vi "Compare pattern (SubVI).vi"(8 "error in":errorcluster, 9 "divider":sgl=1.6, 10 "Angle (degrees)":sgl format="%.2f", 11 "Pattern classes":i32[](array[numeric])) -> (0 "error out":errorcluster, 1 "Number of Matches":i32, 2 "Calibrated Matches":T1[](array[typedef]) {"Correlation Score" format="%.2f"; "Target Template Curve Score" format="%.2f"; "Template Target Curve Score" format="%.2f"; "Bounding Box"."y" format="%.2f"; "Bounding Box"."x" format="%.2f"; "Position"."y" format="%.2f"; "Position"."x" format="%.2f"; "Score" format="%.2f"; "Scale" format="%.2f"; "Angle" format="%.2f"; "Occlusion %" format="%.2f"}, 3 "Pattern":i32, 4 "pattern match":bool)   [LabVIEW 2017]
uses:
  <vilib>/vision/Pattern Matching.llb/IMAQ GM Match Report.ctl
  <vilib>/userdefined/High Color/IMAQdx.ctl
  <vilib>/vision/NI_Vision_Development_Module.lvlib
  <vilib>/vision/driver/NI_Vision_Acquisition_Software.lvlib
panel:
  out "x0":i32
  out "y0":i32
  in  "ROI":T2={"Global Rectangle"=[109, 72, 345, 284], "Contours"=[{"ID"=enum."External", "Type"=3, "Coordinates"=[109, 72, 345, 284]}]} {"Contours"."Type" items=["No Selection", "Point", "Line", "Rectangle", "Oval", "Polygon", "Freehand Region", "Annulus", "Unused2", "Unused3", "Broken Line", "Freehand Line", "Rotated Rectangle"]}
  out "Scale":sgl
  out "x1":i32
  out "y1":i32
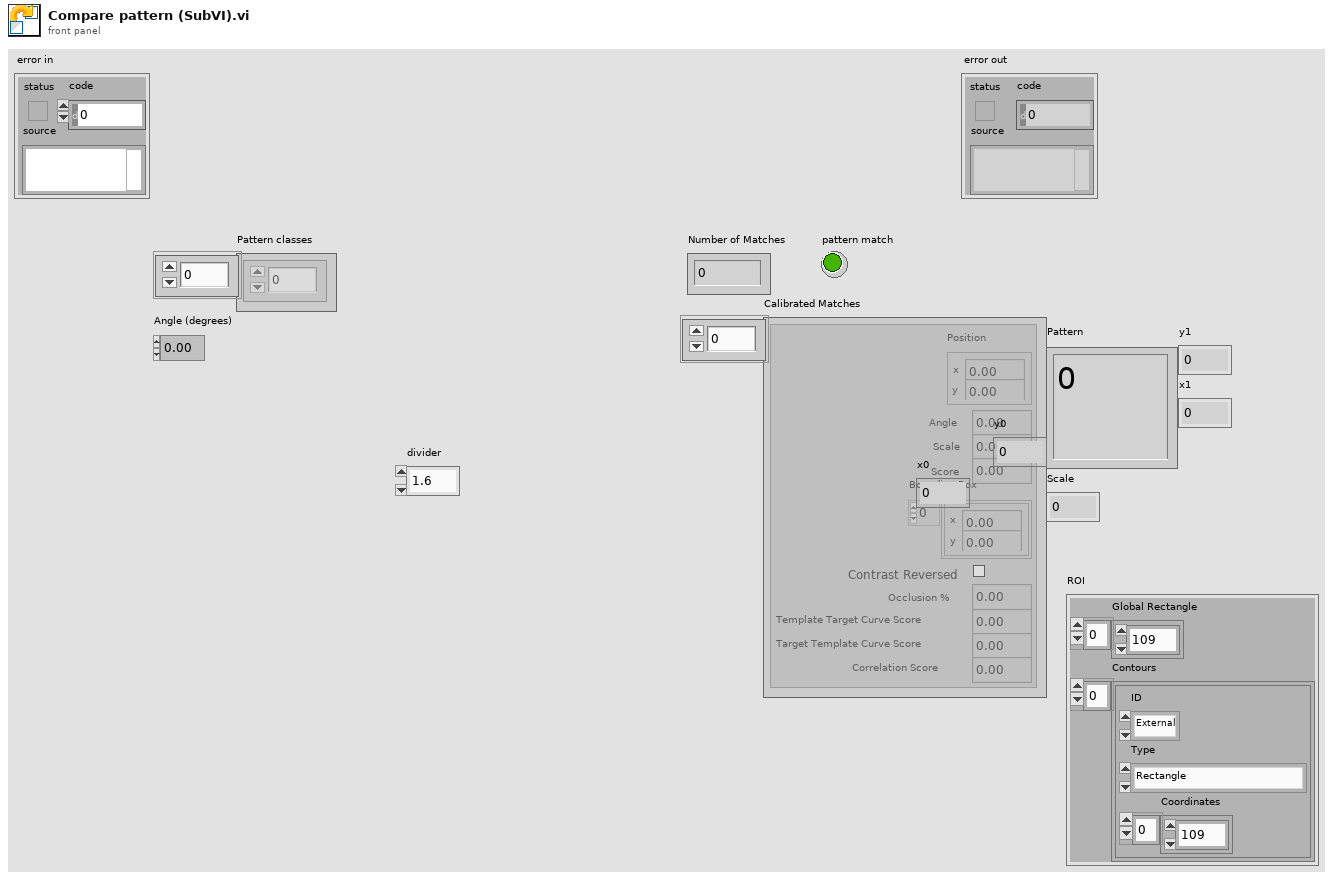
[diagram p1: front panel]
types:
  T1 = typedef "IMAQ GM Match Report.ctl" = cluster{"Position":cluster{"x":sgl, "y":sgl}, "Angle":sgl, "Scale":sgl, "Score":sgl, "Bounding Box":cluster{"x":sgl, "y":sgl}[], "Contrast Reversed":bool, "Occlusion %":sgl, "Template Target Curve Score":sgl, "Target Template Curve Score":sgl, "Correlation Score":sgl}
  T2 = cluster{"Global Rectangle":i32[], "Contours":cluster{"ID":enum32{"External", "Internal"}, "Type":u32, "Coordinates":i32[]}[]}
  T3 = typedef "IMAQdx.ctl" = refnum<k21>
  T4 = typedef "IMAQ Image.ctl" = refnum<image>
  T5 = cluster{"ID":enum32{"External", "Internal"}, "Type":u32, "Coordinates":i32[]}[]
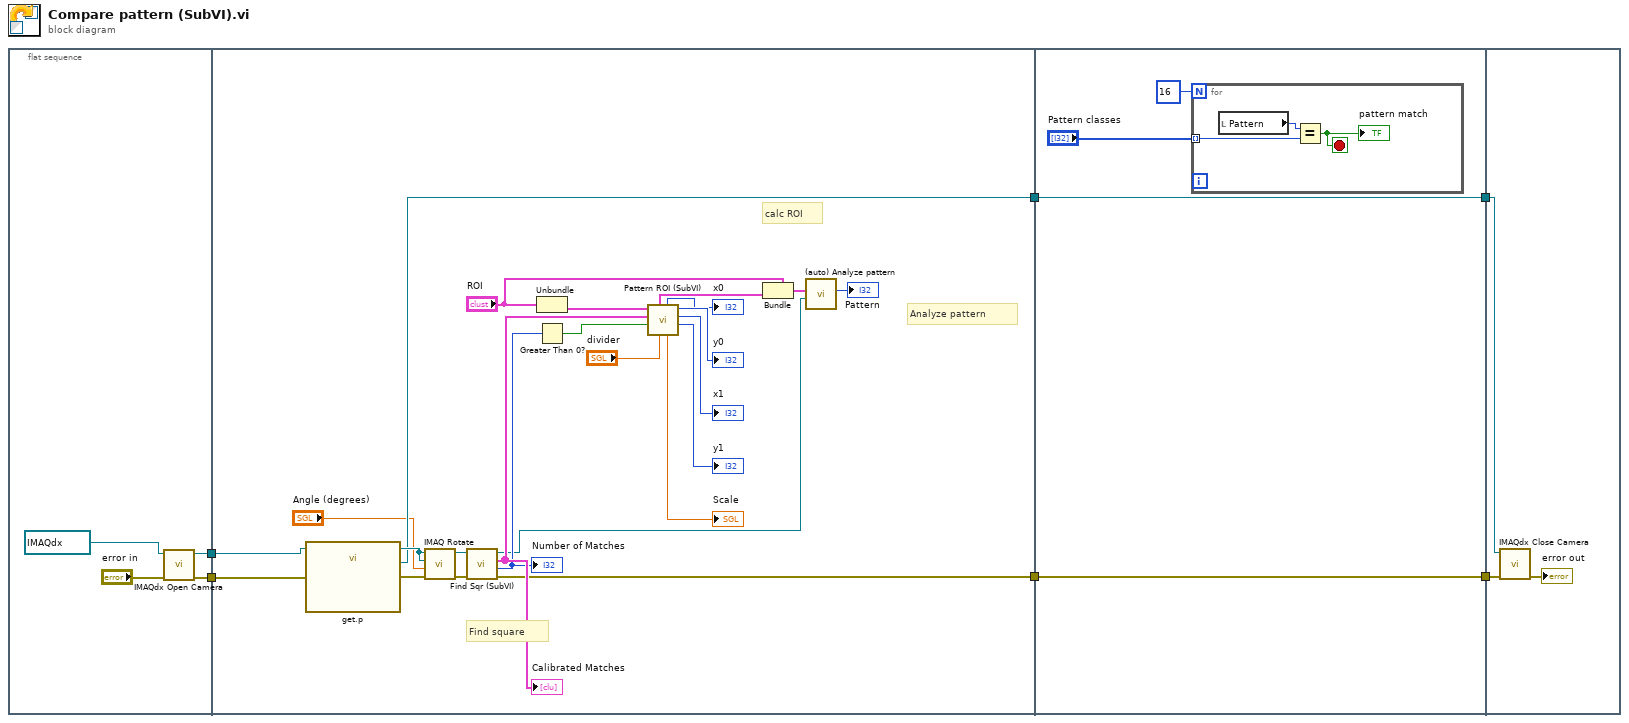
[diagram p0: block diagram]
diagram:
  n1 = flat-sequence {
    tunnel: [w8] -> w6
    tunnel: [w9] -> w5
    tunnel: w6 -> [w15]
    tunnel: w5 -> [w14]
    tunnel: [w13] -> w4
    tunnel: [w11] -> w2
    tunnel: w4 -> [w38]
    tunnel: [w38] -> w3
    tunnel: w2 -> [w35]
    tunnel: [w35] -> w1
    tunnel: w3 -> [w44]
    tunnel: w1 -> [w43]
    frame #0 {
      n2 = call <vilib>:"IMAQdx Open Camera.vi"("error in"="error in", "Session In"=T3 "cam0") -> ("error out"=w9:errorcluster, "Session Out"=w8:T3)  [unwired: 8 in]
    }
    frame #1 {
      # "calc ROI"
      # "Analyze pattern"
      # "Find square"
      n3 = call "get.p.vi"("Session in"=w15, "error in"=w14) -> ("Image Out"=w33:T4, "Session Out"=w13:T3, "error out"=w34:errorcluster)  [unwired: 23 in]
      n4 = call "IMAQ Rotate"("error in (no error)"=w34, "Angle (degrees)"="Angle (degrees)", "Image Dst"=w33, "Image Src"=w33) -> ("error out"=w31:errorcluster, "Image Dst Out"=w32:T4)  [unwired: 6 in]
      n5 = call "Find Sqr (SubVI).vi"("error in (no error)"=w31, "Refnum in"=w32) -> ("error out"=w11:errorcluster, "Number of Matches (Geometric Matching 1)"=w23:i32, "Calibrated Matches (Geometric Matching 1)"=w24:T1[], "Refnum out"=w16:T4)  [unwired: 6 in]
      "Number of Matches" <- w23
      "Calibrated Matches" <- w24
      n6 = Unbundle("ROI") -> ("Contours"=w25:T5)  [unwired: 1 out]
      n7 = Greater Than 0?(x=w23) -> (x > 0?=w22:bool)
      n8 = call "Pattern ROI (SubVI).vi"("divider"="divider", "number of matches"=w22, "Calibrated Matches (Geometric Matching 1)"=w24, "Contours in"=w25) -> ("y1"=→"y1":i32, "x1"=→"x1":i32, "y0"=→"y0":i32, "Scale"=→"Scale":sgl, "x0"=→"x0":i32, "Contours out"=w18:T5)  [unwired: 2 in]
      n9 = Bundle(cluster="ROI", "Contours"=w18) -> (w17:T2)  [unwired: 1 in]
      n10 = call "(auto) Analyze pattern.vi"("Image In"=w16, "ROI Descriptor (Image Mask 1)"=w17) -> ("Pattern"=→"Pattern":i32)  [unwired: 7 in, 2 out]
    }
    frame #2 {
      n11 = for {
        N: 16 -> [_]
        tunnel: "Pattern classes" -> [w40] mode=indexing
        stop <- w39 stop-if-true
        n12 = local read "Pattern"() -> (w41:i32)
        n13 = Equal?(x=w41, y=w40) -> (x = y?=w39:bool)
        "pattern match" <- w39
      }
    }
    frame #3 {
      n14 = call <vilib>:"IMAQdx Close Camera.vi"("error in"=w43, "Session In"=w44) -> ("error out"=→"error out":errorcluster)  [unwired: 9 in]
    }
  }
